vi "Position-write (SubVI).vi"(6 "Position":i16(knob) max=1023 scale=0.0..4096.0, 9 "ID":u8) -> (3 "result string":string)   [LabVIEW 2017]
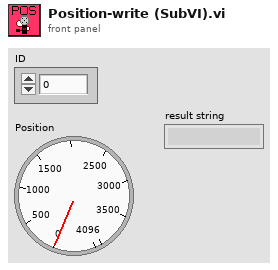
[diagram p1: front panel]
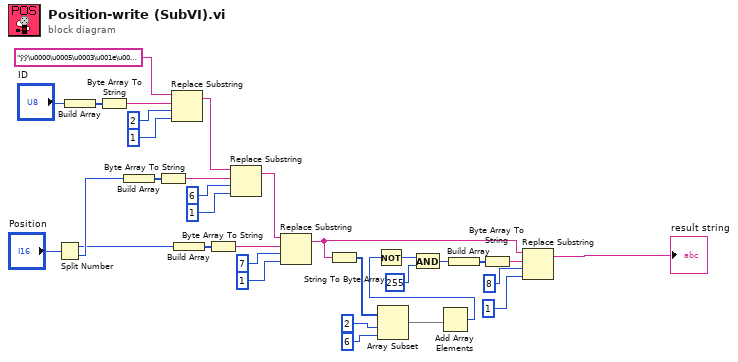
[diagram p0: block diagram]
diagram:
  n1 = Split Number(x="Position") -> (hi(x)=w31:u8, lo(x)=w32:u8)
  n2 = Build Array("ID") -> (w20:u8[])
  n3 = Byte Array To String(unsigned byte array=w20) -> (string=w22:string)
  n4 = Build Array(w32) -> (w16:u8[])
  n5 = Byte Array To String(unsigned byte array=w16) -> (string=w17:string)
  n6 = Replace Substring(2:1 ("length (len. of substring)"), 3:2 ("offset (0)"), 4:w22, 5:"ÿÿ\u0000\u0005\u0003\u001e\u0000\u0000\u0000" ("string")) -> (1:w13:string)  [unwired: 1 out]
  n7 = Build Array(w31) -> (w27:u8[])
  n8 = Byte Array To String(unsigned byte array=w27) -> (string=w28:string)
  n9 = Replace Substring(2:1 ("length (len. of substring)"), 3:6 ("offset (0)"), 4:w17, 5:w13) -> (1:w29:string)  [unwired: 1 out]
  n10 = Replace Substring(2:1 ("length (len. of substring)"), 3:7 ("offset (0)"), 4:w28, 5:w29) -> (1:w30:string)  [unwired: 1 out]
  n11 = String To Byte Array(string=w30) -> (unsigned byte array=w5:u8[])
  n12 = Array Subset(array=w5, index=2, length=6) -> (w2:u8[])
  n13 = Add Array Elements(numeric array=w2) -> (sum=w1:u8)
  n14 = Not(x=w1) -> (.not. x?=w12:u8)
  n15 = And(x=w12, y=u8 255) -> (x .and. y?=w6:u8)
  n16 = Build Array(w6) -> (w9:u8[])
  n17 = Byte Array To String(unsigned byte array=w9) -> (string=w10:string)
  n18 = Replace Substring(2:1 ("length (len. of substring)"), 3:8 ("offset (0)"), 4:w10, 5:w30) -> (1:→"result string":string)  [unwired: 1 out]
